vi "Parameter Set (No Objects).vi"(8 "error in (no error)":errorcluster, 11 "Cluster In":T2={"Wavelength"=0.0, "AVG"=0, "Range"=0, "Backlight"=0, "Beeper"=0, "Zero"=0, "Local Lockout"=0, "ATTN"=0, "Run/Stop"=0, "Units"=0, "Averaging Time"=0.5, "Averaging"=FALSE, "Most Recent Power"=5.5, "Filter"=1} {"AVG" items=["Slow"=1, "Medium"=2, "Fast"=3]; "Range" items=["Auto", "Lowest", "2", "3", "4", "5", "6", "7", "Highest"]; "Backlight" items=["Off", "Low", "High"]; "Beeper" items=["Off", "On"]; "Zero" items=["Off", "On"]; "Local Lockout" items=["Off", "On"]; "ATTN" items=["Off", "On"]; "Run/Stop" items=["Stop", "Run"]; "Units" items=["W"=1, "dB"=2, "dBm"=3, "REL"=4]; "Filter" items=["Orange"=1, "Green"=2, "Yellow"=3]}) -> (0 "error out":errorcluster, 3 "Cluster Out":T2={"Wavelength"=0.0, "AVG"=0, "Range"=0, "Backlight"=0, "Beeper"=0, "Zero"=0, "Local Lockout"=0, "ATTN"=0, "Run/Stop"=0, "Units"=0, "Averaging Time"=0.5, "Averaging"=FALSE, "Most Recent Power"=5.5, "Filter"=1} {"AVG" items=["Slow"=1, "Medium"=2, "Fast"=3]; "Range" items=["Auto", "Lowest", "2", "3", "4", "5", "6", "7", "Highest"]; "Backlight" items=["Off", "Low", "High"]; "Beeper" items=["Off", "On"]; "Zero" items=["Off", "On"]; "Local Lockout" items=["Off", "On"]; "ATTN" items=["Off", "On"]; "Run/Stop" items=["Stop", "Run"]; "Units" items=["W"=1, "dB"=2, "dBm"=3, "REL"=4]; "Filter" items=["Orange"=1, "Green"=2, "Yellow"=3]})   [LabVIEW 2012]
doc: "Opens pop-up window for changing Newport 1830-C parameter settings within another control panel."
uses:
  Newport 1830-C/Public/Filters.ctl
  Global/GPIB Numbers.vi
panel:
  in  "Filter":T1=1 items=["Orange"=1, "Green"=2, "Yellow"=3]
  out "Error":bool
  in  "stop":bool
  in  "R2C":bool
  in  "Averaging Time":dbl[unit]=0.5
  in  "Averaging?":bool
  in  "Local Lockout (0:1)":u32(ring) items=["Off", "On"]
  in  "ATTN (0:1)":u32(ring)=1 items=["Off", "On"]
  in  "Run/Stop (1:0)":u32(ring)=1 items=["Stop", "Run"]
  in  "AVG (1:3)":u32(ring)=2 items=["Slow"=1, "Medium"=2, "Fast"=3]
  in  "Units (1:4)":u32(ring)=1 items=["W"=1, "dB"=2, "dBm"=3, "REL"=4]
  in  "Zero (0:1)":u32(ring) items=["Off", "On"]
  in  "Beeper (0:1)":u32(ring) items=["Off", "On"]
  in  "Backlight (0:2)":u32(ring)=1 items=["Off", "Low", "High"]
  in  "Range (0-Auto,1:8)":u32(ring) items=["Auto", "Lowest", "2", "3", "4", "5", "6", "7", "Highest"]
  in  "Wavelength (nnnn)":dbl[unit]=8.210000000000001e-07
  in  "Set":bool
  # "Only use Watts with LPC!"
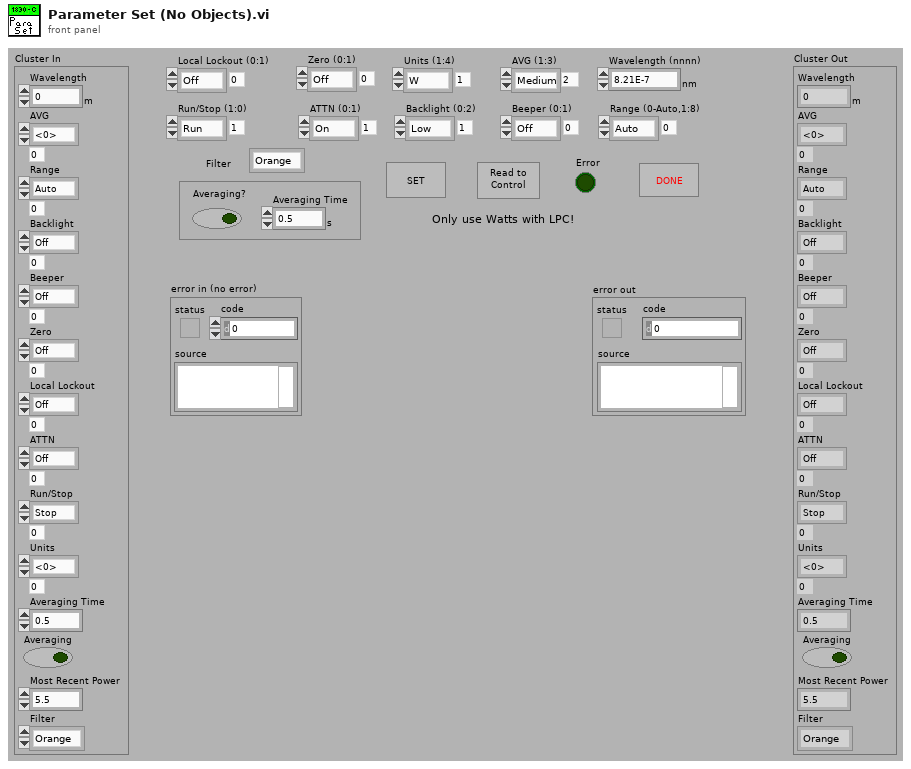
[diagram p1: front panel]
types:
  T1 = typedef "Filters.ctl" = u16
  T2 = cluster{"Wavelength":dbl[unit], "AVG":u16, "Range":u16, "Backlight":u16, "Beeper":u16, "Zero":u16, "Local Lockout":u16, "ATTN":u16, "Run/Stop":u16, "Units":u16, "Averaging Time":dbl, "Averaging":bool, "Most Recent Power":dbl, "Filter":T1}
  T3 = typedef "GPIB Type Def.ctl" = cluster{"Name":string, "bus":dbl, "GPIB":dbl, "GPIB as string":string, "byte":i32, "VISA Resource Name":refnum<visa-resource-name>}
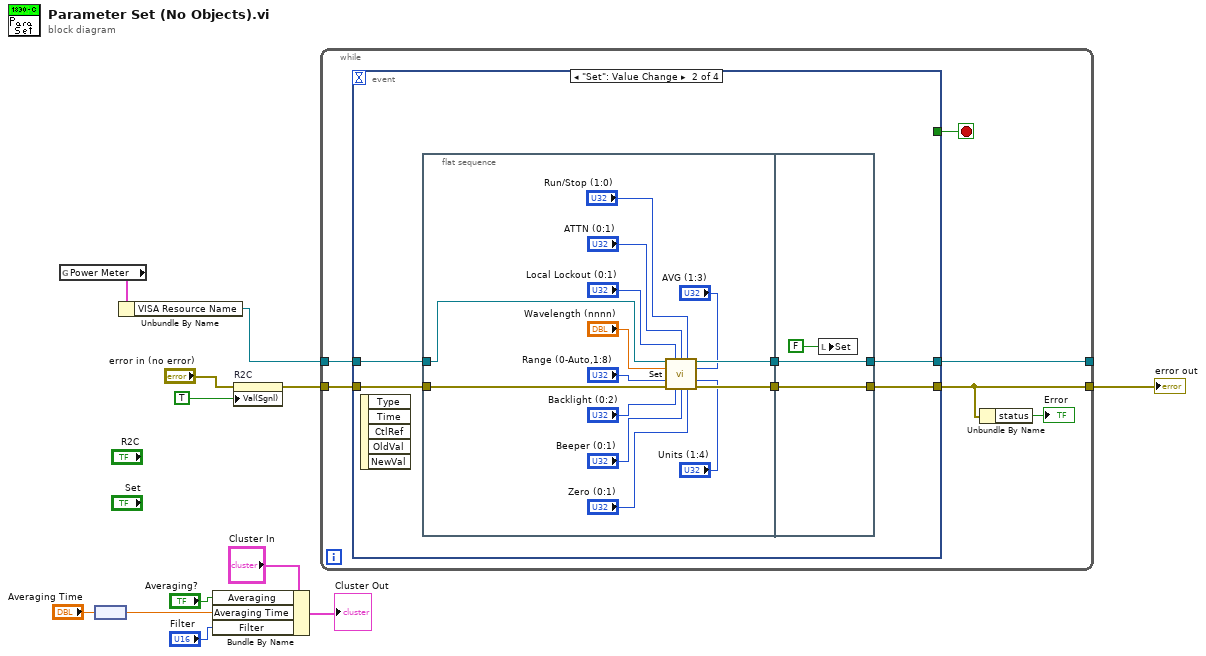
[diagram p0: block diagram]
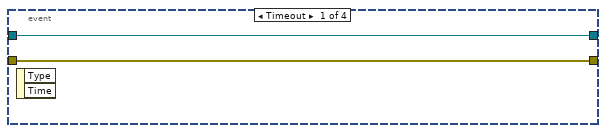
[diagram p2: hidden frame]
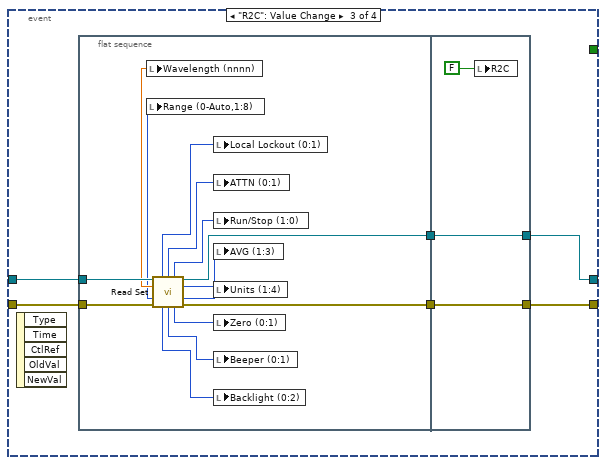
[diagram p3: hidden frame]
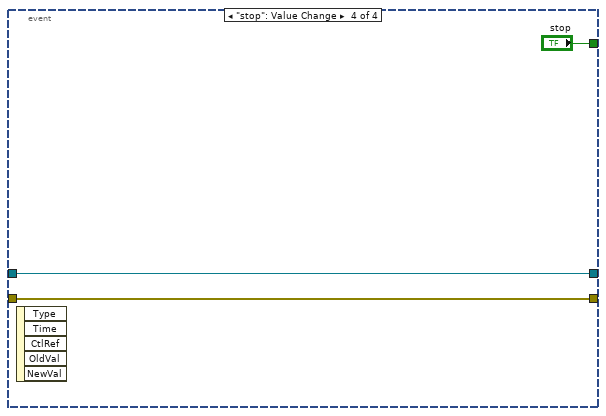
[diagram p4: hidden frame]
diagram:
  n1 = global read "GPIB Numbers.vi" "Power Meter"() -> (w3:T3)
  n2 = node("Averaging Time") -> (w10:dbl)
  n3 = Unbundle By Name(w3) -> ("VISA Resource Name"=w2:refnum<visa-resource-name>)
  n4 = Bundle By Name(cluster="Cluster In", "Averaging"="Averaging?", "Averaging Time"=w10, "Filter"="Filter") -> (→"Cluster Out":T2)
  n5 = property on="R2C" class="Bool (strict)"(error in="error in (no error)", "Val(Sgnl)"=TRUE ("Value (Signaling)")) -> (error out=w8:errorcluster)  [unwired: 1 in, 1 out]
  n6 = while {
    tunnel: w8 -> [w18]
    tunnel: w2 -> [w17]
    tunnel: [w16] -> _
    tunnel: [w14] -> w5
    stop <- w15 stop-if-true
    n7 = event shown="[1] \"Set\": Value Change" {
      selector: _ -> [_ _ _ _]
      dyn-events: _ -> [_ _ _ _]
      timeout: _ -> [_ _ _ _]
      tunnel: [w20 w26 w48 w69] -> w16
      tunnel: w18 -> [w19 w25 w47 w68]
      tunnel: [w19 w24 w46 w68] -> w14
      tunnel: w17 -> [w20 w23 w49 w69]
      tunnel: [_ _ _ "stop"] -> w15
      event Timeout {
        n8 = event-data() -> ()  [unwired: 1 in, 2 out]
      }
      event "Set": Value Change {
        n9 = event-data() -> ()  [unwired: 1 in, 5 out]
        n10 = flat-sequence {
          tunnel: [w40] -> w22
          tunnel: w25 -> [w37]
          tunnel: [w33] -> w21
          tunnel: w23 -> [w27]
          tunnel: [w42] -> w26
          tunnel: w22 -> [w42]
          tunnel: [w41] -> w24
          tunnel: w21 -> [w41]
          frame #0 {
            n11 = call "Set.vi"("VISA resource name"=w27, "Local Lockout (0:1)"="Local Lockout (0:1)", "ATTN (0:1)"="ATTN (0:1)", "Run/Stop (1:0)"="Run/Stop (1:0)", "Wavelength (nnnn)"="Wavelength (nnnn)", "AVG (1:3)"="AVG (1:3)", "Range (0-Auto,1:8)"="Range (0-Auto,1:8)", "Units (1:4)"="Units (1:4)", "error in (no error)"=w37, "Backlight (0:2)"="Backlight (0:2)", "Beeper (0:1)"="Beeper (0:1)", "Zero (0:1)"="Zero (0:1)") -> ("VISA resource name out"=w40:refnum<visa-resource-name>, "error out"=w33:errorcluster)  [unwired: 2 in]
          }
          frame #1 {
            n12 = local write "Set"(FALSE ("Set")) -> ()
          }
        }
      }
      event "R2C": Value Change {
        n13 = event-data() -> ()  [unwired: 1 in, 5 out]
        n14 = flat-sequence {
          tunnel: w49 -> [w63]
          tunnel: [w62] -> w45
          tunnel: w47 -> [w61]
          tunnel: [w60] -> w44
          tunnel: [w65] -> w48
          tunnel: w45 -> [w65]
          tunnel: [w64] -> w46
          tunnel: w44 -> [w64]
          frame #0 {
            n15 = call "Read Set.vi"("VISA resource name"=w63, "error in (no error)"=w61) -> ("Local Lockout"=w59:u32, "ATTN"=w58:u32, "Run/Stop"=w57:u32, "VISA resource name out"=w62:refnum<visa-resource-name>, "Wavelength (nnnn)"=w51:dbl[unit], "AVG"=w56:u32, "Range (1:8)"=w50:u32, "Units"=w55:u32, "Backlight"=w54:u32, "Beeper"=w53:u32, "Zero"=w52:u32, "error out"=w60:errorcluster)  [unwired: 2 in]
            n16 = local write "Wavelength (nnnn)"(w51) -> ()
            n17 = local write "Range (0-Auto,1:8)"(w50) -> ()
            n18 = local write "Local Lockout (0:1)"(w59) -> ()
            n19 = local write "ATTN (0:1)"(w58) -> ()
            n20 = local write "Run/Stop (1:0)"(w57) -> ()
            n21 = local write "AVG (1:3)"(w56) -> ()
            n22 = local write "Units (1:4)"(w55) -> ()
            n23 = local write "Zero (0:1)"(w52) -> ()
            n24 = local write "Beeper (0:1)"(w53) -> ()
            n25 = local write "Backlight (0:2)"(w54) -> ()
          }
          frame #1 {
            n26 = local write "R2C"(FALSE ("R2C")) -> ()
          }
        }
      }
      event "stop": Value Change {
        n27 = event-data() -> ()  [unwired: 1 in, 5 out]
      }
    }
    n28 = Unbundle By Name(w14) -> ("status"=→"Error":bool)
  }
  "error out" <- w5
